vi "K2182A_Queue_Commands.vi"(1 "K2182A Control":T1, 3 "Queue in":refnum<queue>) -> (0 "New Status":T1)   [LabVIEW 2019]
uses:
  K2182A/K2812A_control.ctl
  Equipment/Keithley 622x/Configure/2182 -A/Low Level/Typedefs/KE2182 -- Voltage Ranges.ctl
  Equipment/Keithley 622x/Keithley 622x.lvlib
panel:
  # "K 2182A"
  # "K 2182A"
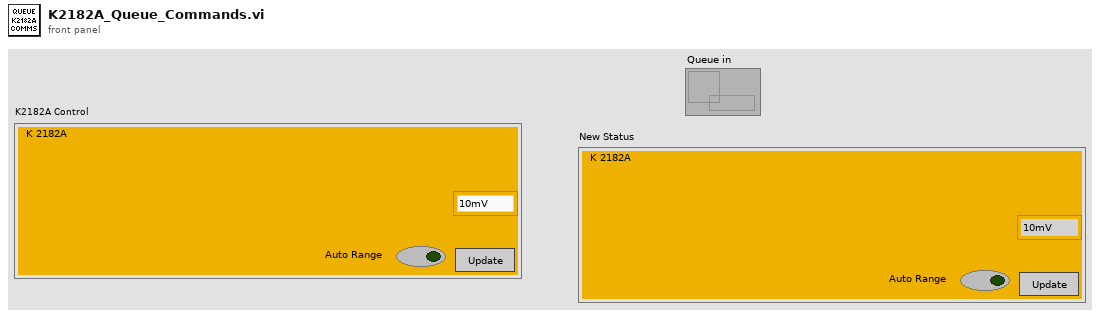
[diagram p1: front panel]
types:
  T1 = typedef "K2812A_control.ctl" = cluster{"Update":bool, "Range selector":T2, "Auto Range":bool}
  T2 = typedef "Keithley 622x.lvlib/KE2182 -- Voltage Ranges.ctl" = enum16{"10mV", "100mV", "1V", "10V", "100V"}
  T3 = cluster{"Update":bool, "Range selector":bool, "Auto Range":bool}
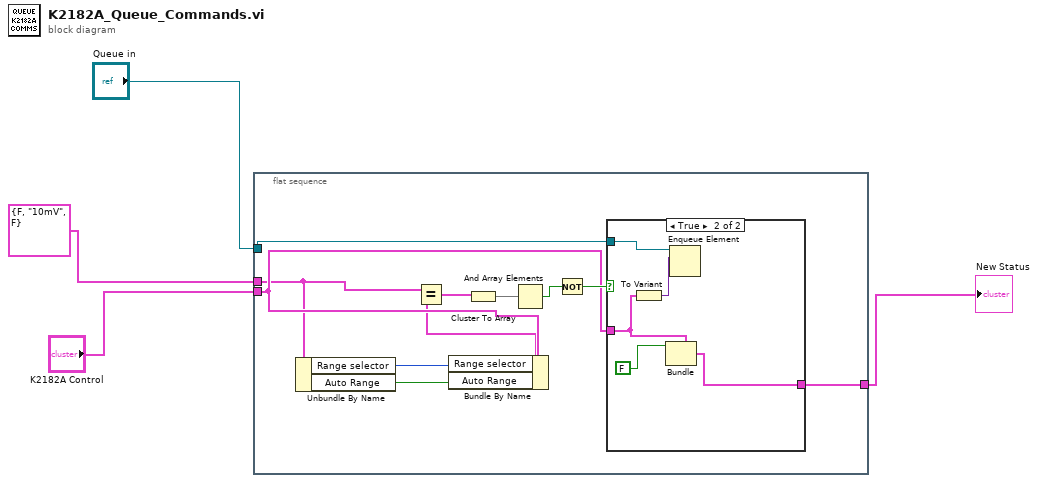
[diagram p0: block diagram]
diagram:
  n1 = flat-sequence {
    tunnel: "Queue in" -> [w15]
    tunnel: "K2182A Control" -> [w9]
    tunnel: T1 {"Update"=FALSE, "Range selector"=enum."10mV", "Auto Range"=FALSE} ("K2182A Cluster 2") -> [w8]
    tunnel: [w10] -> w2
    frame #0 {
      n2 = Unbundle By Name(w8) -> ("Range selector"=w6:T2, "Auto Range"=w5:bool)
      n3 = Bundle By Name(cluster=w9, "Range selector"=w6, "Auto Range"=w5) -> (w7:T1)
      n4 = Equal?(x=w8, y=w7) -> (x = y?=w11:T3)
      n5 = Cluster To Array(cluster=w11) -> (array=w14:bool[])
      n6 = And Array Elements(Boolean array=w14) -> (logical AND=w13:bool)
      n7 = Not(x=w13) -> (.not. x?=w12:bool)
      n8 = case shown="True" w12 {
        tunnel: w15 -> [_ w21]
        tunnel: w9 -> [w16 w19]
        tunnel: [w16 w18] -> w10
        frame False {
        }
        frame True {
          n9 = To Variant(anything=w19) -> (Variant=w20:variant)
          n10 = Bundle(cluster=w19, "Update"=FALSE) -> (w18:T1)  [unwired: 2 in]
          n11 = Enqueue Element(queue=w21, element=w20) -> ()  [unwired: 2 in, 3 out]
        }
      }
    }
  }
  "New Status" <- w2
